vi "Wave2D_Check Input.vi"(0 "F(t, x, y)":dbl[][][](array[numeric]), 1 "Initial Value":dbl[][](array[numeric]), 2 "Initial Derivative":dbl[][](array[numeric]), 5 "k":dbl=1.0, 7 "a":dbl, 9 "Domain":T2={"t"={"initial t"=0.0, "final t"=1.0, "# of t-points"=11}, "x"={"start x"=0.0, "end x"=1.0, "# of x-points"=11}, "y"={"start y"=0.0, "end y"=1.0, "# of y-points"=11}}, 11 "error in (no error)":errorcluster, 12 "Boundary Condition":cluster{"type":T1, "Value":dbl[][]}[](array[cluster]) {"type" items=["Dirichlet", "Neumann"]}) -> (15 "error out":errorcluster)   [LabVIEW 2020, in "NI_PDE.lvlib"]
uses:
  <vilib>/gmath/NI_PDE.lvlib
  <vilib>/gmath/pde.llb/Common/PDE_BC Type.ctl
  <vilib>/gmath/pde.llb/Common/PDE_Error.ctl
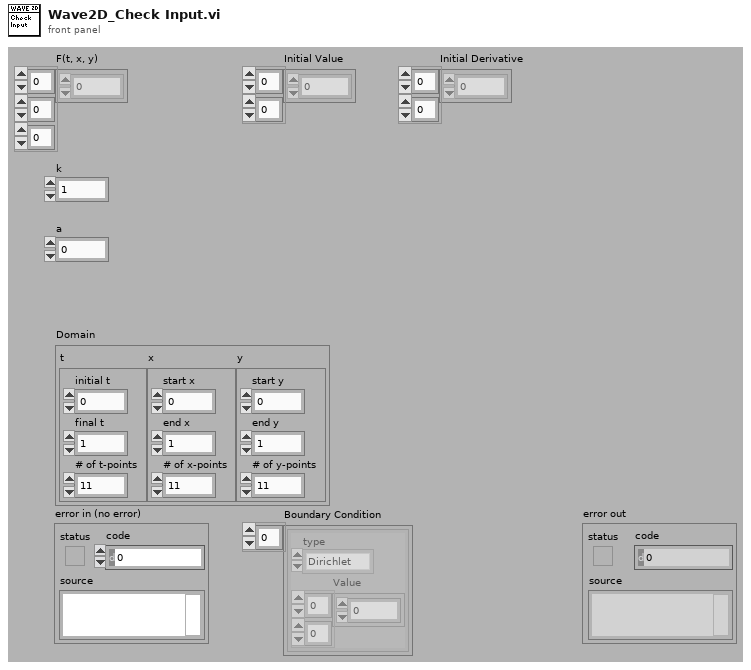
[diagram p1: front panel]
types:
  T1 = typedef "NI_PDE.lvlib/PDE_BC Type.ctl" = i32
  T2 = cluster{"t":cluster{"initial t":dbl, "final t":dbl, "# of t-points":i32}, "x":cluster{"start x":dbl, "end x":dbl, "# of x-points":i32}, "y":cluster{"start y":dbl, "end y":dbl, "# of y-points":i32}}
  T3 = typedef "NI_PDE.lvlib/PDE_Error.ctl" = enum16{"No Error", "k is zero", "End point <= start point", "# of time steps < 2", "# of spatial points < 3", "# of grid < 1 for FEM", "# of boundary < 3 for FEM", "Incompatible RHS size", "Incompatible BC size", "Incompatible IC size", "PDE class conflict", "RHS class conflict", "Domain class conflict", "BC class conflict", "IC class conflict"}
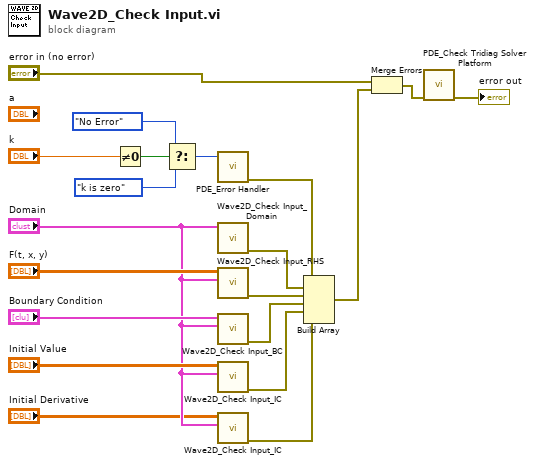
[diagram p0: block diagram]
diagram:
  n1 = Not Equal To 0?(x="k") -> (x != 0?=w20:bool)
  n2 = Select(t=PDE_Error."No Error" ("PDE error"), s=w20, f=PDE_Error."k is zero" ("PDE error")) -> (s? t:f=w17:T3)
  n3 = call <vilib>:"PDE_Error Handler.vi"("PDE error"=w17) -> ("error out"=w9:errorcluster)  [unwired: 1 in, 9 out]
  n4 = call <vilib>:"Wave2D_Check Input_Domain.vi"("Domain"="Domain") -> ("error out"=w1:errorcluster)  [unwired: 1 in, 9 out]
  n5 = call <vilib>:"Wave2D_Check Input_RHS.vi"("Domain"="Domain", "F(t, x, y)"="F(t, x, y)") -> ("error out"=w2:errorcluster)  [unwired: 1 in, 8 out]
  n6 = call <vilib>:"Wave2D_Check Input_BC.vi"("Domain"="Domain", "Boundary Condition"="Boundary Condition") -> ("error out"=w8:errorcluster)  [unwired: 1 in, 8 out]
  n7 = call <vilib>:"Wave2D_Check Input_IC.vi"("Domain"="Domain", "Initial Value"="Initial Value") -> ("error out"=w7:errorcluster)  [unwired: 1 in, 8 out]
  n8 = call <vilib>:"Wave2D_Check Input_IC.vi"("Domain"="Domain", "Initial Value"="Initial Derivative") -> ("error out"=w6:errorcluster)  [unwired: 1 in, 8 out]
  n9 = Build Array(w9, w1, w2, w8, w7, w6) -> (w5:errorcluster[])
  n10 = Merge Errors("error in (no error)", w5) -> (w4:errorcluster)
  n11 = call <vilib>:"PDE_Check Tridiag Solver Platform.vi"("error in (no error)"=w4) -> ("error out"=→"error out":errorcluster)  [unwired: 10 out]
